vi "HasProperty.vi"(8 "error in (no error)":errorcluster, 10 "Property":string, 11 "CSSProperties in":refnum<class "CSSProperties.lvclass">) -> (0 "error out":errorcluster, 2 "Exists?":bool, 3 "CSSProperties out":refnum<class "CSSProperties.lvclass">)   [LabVIEW 2019, in "CSSProperties.lvclass"]
uses:
  CSSProperties.lvclass
  CSSProperties.lvclass/CSSProperties.ctl
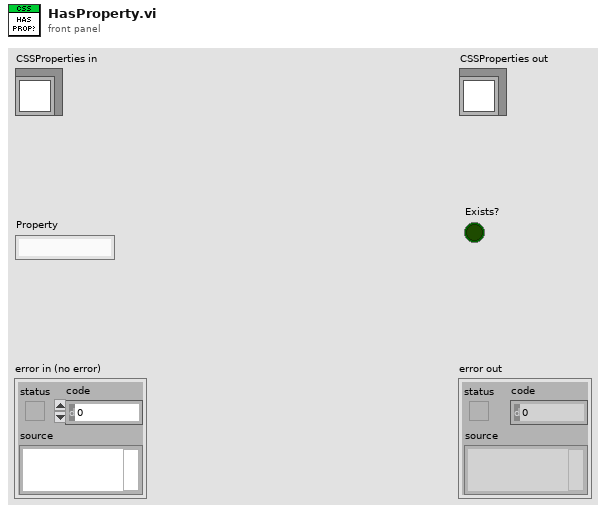
[diagram p1: front panel]
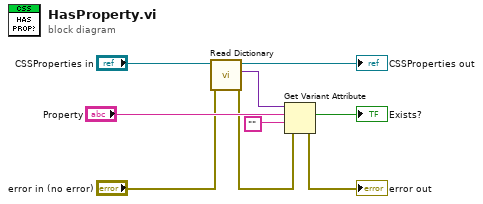
[diagram p0: block diagram]
diagram:
  n1 = call "Read Dictionary.vi"("error in (no error)"="error in (no error)", "CSSProperties in"="CSSProperties in") -> ("error out"=w3:errorcluster, "Dictionary"=w7:variant, "CSSProperties out"=→"CSSProperties out":refnum<class "CSSProperties.lvclass">)  [unwired: 7 in]
  n2 = Get Variant Attribute(Variant=w7, name="Property", default value (empty Variant)="", error in=w3) -> (found=→"Exists?":bool, error out=→"error out":errorcluster)  [unwired: 2 out]
